vi "NewObj.vi"(8 "error in (no error)":errorcluster, 11 "reference in":refnum<class "Object_Editor.lvclass">) -> (0 "error out":errorcluster, 3 "reference out":refnum<class "Object_Editor.lvclass">)   [LabVIEW 2022 SP3, in "Object_Editor.lvlib" / "Object_Editor.lvclass"]
uses:
  Object_Editor.lvclass
  Components/ViPER.lvlibp/ViPER.lvclass
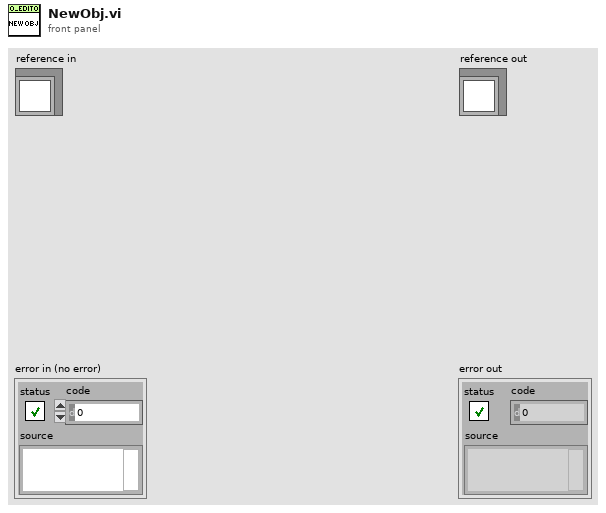
[diagram p1: front panel]
types:
  T1 = typedef "Object_Editor.lvlib/Object_Editor.lvclass/ObjectAttributes.ctl" = cluster{"Config":T2, "Tree":refnum<vi>, "Mod_Bit":bool, "File_Path":path, "Object":refnum<class "ViPER.lvclass">}
  T2 = typedef "Object_Editor.lvlib/Object_Editor.lvclass/Config.ctl" = cluster{"default":string}
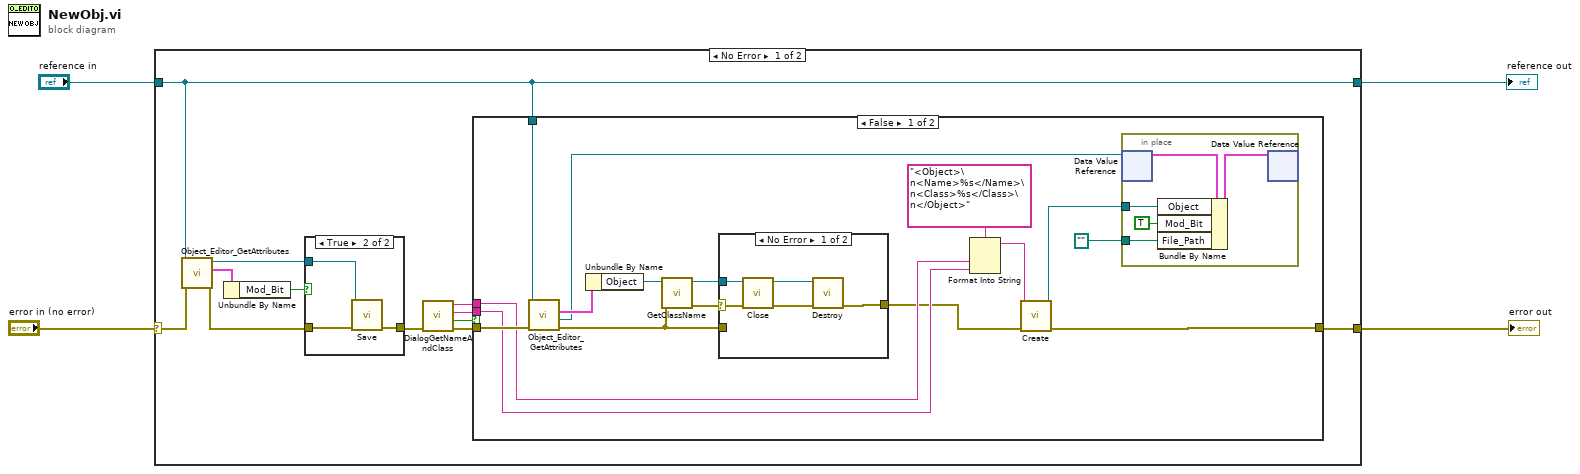
[diagram p0: block diagram]
diagram:
  n1 = case shown="No Error" "error in (no error)" {
    selector: "error in (no error)" -> [w11 w50]
    tunnel: [w16 w50] -> w1
    tunnel: [w10 w49] -> w2
    tunnel: "reference in" -> [w10 w49]
    frame No Error {
      n2 = call "Object_Editor_GetAttributes.vi"("error in (no error)"=w11, "reference in"=w10) -> ("error out"=w9:errorcluster, "Data"=w7:T1, "reference out"=w5:refnum<class "Object_Editor.lvclass">)  [unwired: 6 in, 1 out]
      n3 = Unbundle By Name(w7) -> ("Mod_Bit"=w6:bool)
      n4 = case shown="True" w6 {
        tunnel: w9 -> [w17 w20]
        tunnel: [w17 w19] -> w8
        tunnel: w5 -> [_ w18]
        frame False {
        }
        frame True {
          n5 = call "Save.vi"("error in (no error)"=w20, "reference in"=w18) -> ("error out"=w19:errorcluster)  [unwired: 8 in, 1 out]
        }
      }
      n6 = call "DialogGetNameAndClass.vi"("error in (no error)"=w8) -> ("error out"=w15:errorcluster, "Cancelled"=w14:bool, "Class"=w13:string, "Name"=w12:string)  [unwired: 7 in]
      n7 = case shown="False" w14 {
        tunnel: w10 -> [w36 _]
        tunnel: [w21 w48] -> w16
        tunnel: w15 -> [w32 w48]
        tunnel: w13 -> [w30 _]
        tunnel: w12 -> [w29 _]
        frame False {
          n8 = call "Object_Editor_GetAttributes.vi"("error in (no error)"=w32, "reference in"=w36) -> ("error out"=w27:errorcluster, "DataRef"=w34:refnum<data-value>, "Data"=w35:T1)  [unwired: 6 in, 1 out]
          n9 = Unbundle By Name(w35) -> ("Object"=w28:refnum<class "ViPER.lvclass">)
          n10 = call "GetClassName.vi"("error in (no error)"=w27, "reference in"=w28) -> ("error out"=w26:errorcluster, "reference out"=w25:refnum<class "ViPER.lvclass">)  [unwired: 7 in, 1 out]
          n11 = case shown="No Error" w26 {
            selector: w26 -> [w46 _]
            tunnel: w25 -> [w45 _]
            tunnel: [w42 w47] -> w22
            tunnel: w27 -> [_ w47]
            frame No Error {
              n12 = call-dynamic "Close.vi"("error in (no error)"=w46, "reference in"=w45) -> ("error out"=w43:errorcluster, "reference out"=w44:refnum<class "ViPER.lvclass">)  [unwired: 8 in]
              n13 = call "Destroy.vi"("error in (no error)"=w43, "reference in"=w44) -> ("error out"=w42:errorcluster)  [unwired: 9 in]
            }
            frame Error {
            }
          }
          n14 = Format Into String(format string="<Object>\n<Name>%s</Name>\n<Class>%s</Class>\n</Object>", w29, w30) -> (resulting string=w24:string)  [unwired: 2 in, 1 out]
          n15 = call "Create.vi"("error in (no error)"=w22, "Config XML"=w24) -> ("error out"=w21:errorcluster, "reference out"=w23:refnum<class "ViPER.lvclass">)  [unwired: 8 in]
          n16 = in-place {
            in-place-border: w23 -> [w39]
            in-place-border: path "" -> [w37]
            n17 = in-place-dvr #1(w34) -> (w41:T1)  [unwired: 1 out]
            n18 = Bundle By Name(cluster=w41, "Object"=w39, "Mod_Bit"=TRUE, "File_Path"=w37) -> (w40:T1)
            n19 = in-place-dvr #1(w40) -> ()  [unwired: 2 out]
          }
        }
        frame True {
        }
      }
    }
    frame Error {
    }
  }
  "error out" <- w1
  "reference out" <- w2
